vi "As XY Projection.vi"(11 "Hailstone in":refnum<class "Hailstone.lvclass">) -> (2 "Trace":refnum<class "Trace.lvclass">)   [LabVIEW 2021, in "Hailstone.lvclass"]
uses:
  Hailstone.lvclass
  Trace/Trace.lvclass
  Hailstone.lvclass/Hailstone.ctl
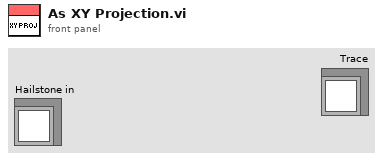
[diagram p1: front panel]
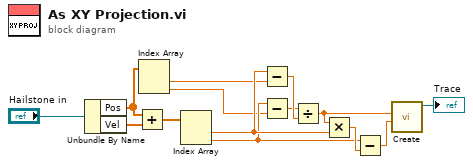
[diagram p0: block diagram]
diagram:
  n1 = Unbundle By Name("Hailstone in") -> ("Pos"=w6:ext[], "Vel"=w5:ext[])
  n2 = Add(x=w6, y=w5) -> (x+y=w7:ext[])
  n3 = Index Array(array=w6) -> (element #1=w8:ext, element #2=w9:ext)  [unwired: 2 in]
  n4 = Index Array(array=w7) -> (element #1=w13:ext, element #2=w12:ext)  [unwired: 2 in]
  n5 = Subtract(x=w13, y=w8) -> (x-y=w11:ext)
  n6 = Subtract(x=w12, y=w9) -> (x-y=w10:ext)
  n7 = Divide(x=w10, y=w11) -> (x/y=w3:ext)
  n8 = Multiply(x=w3, y=w13) -> (x*y=w14:ext)
  n9 = Subtract(x=w12, y=w14) -> (x-y=w2:ext)
  n10 = call "Create.vi"("Offset"=w2, "Slope"=w3) -> ("Trace"=→"Trace":refnum<class "Trace.lvclass">)  [unwired: 8 in, 1 out]
